vi "Main_Basic.vi"() -> ()   [LabVIEW 2021]
doc: "This template is for the Queued Message Handler design pattern.\n\nThe Event Handling Loop generates messages based on user interface actions.\n\nThe Message Handling Loop processes messages generated by the Event Handling Loop, or by other messages. The messages are string values, so new messages can be added easily to the Message Cases case structure in the Message Handling Loop. Each message cluster can also provide an optional value for Message Data, which is a variant that can be converted to whatever message-specific data is required."
uses:
  Controls/Status Lights.ctl
  Controls/UI Data.ctl
  Controls/Timer Actions.ctl
  support/Message Queue/Enqueue Message (Single).vi
  <vilib>/Utility/error.llb/Error Cluster From Error Code.vi
  <vilib>/ErrorRing/Error Ring.xnode
  support/Message Queue/Message Queue.lvlib
  support/User Event - Stop/User Event - Stop.lvlib
panel:
  out "Sampling Active":bool=TRUE
  out "Pressure":dbl(knob) scale=0.0..10.0
  out "Pressure (Bar)":dbl
  out "Sampling State":string
  in  "Start Pressure Logging":bool
  out "Speed Indicator":dbl
  in  "Release Brake":bool
  in  "Retract":bool
  out "Status":T1
  in  "Speed (v)":dbl(knob) scale=0.0..5.0
  out "Status Message":string
  in  "Extend":bool
  in  "Apply Brake":bool
  in  "Exit":bool
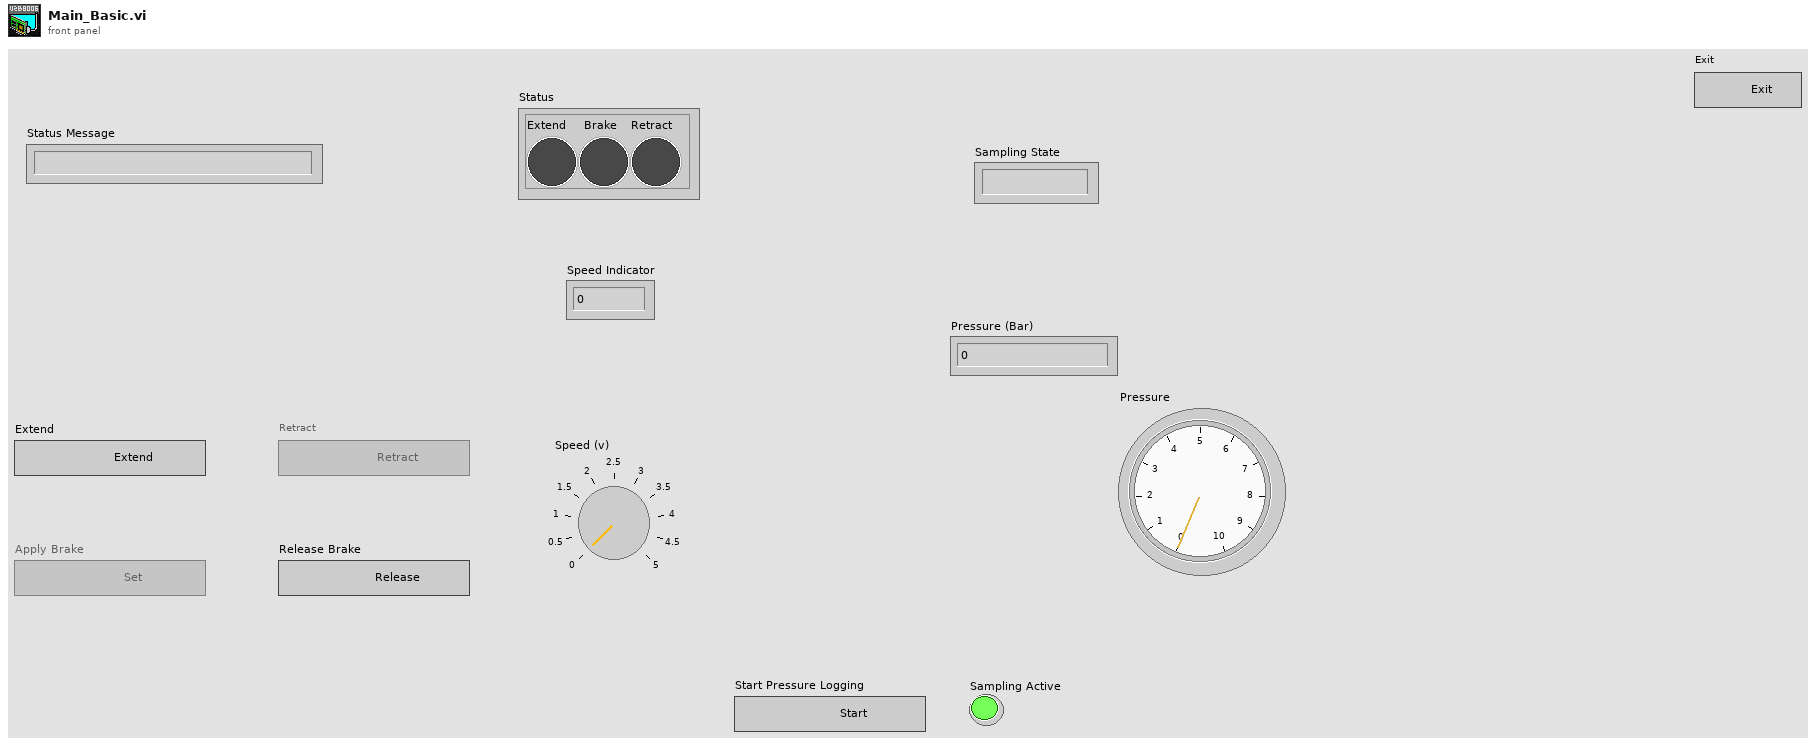
[diagram p1: front panel]
types:
  T1 = typedef "Status Lights.ctl" = cluster{"Extend":bool, "Brake":bool, "Retract":bool}
  T2 = typedef "UI Data.ctl" = cluster{"Sampling State":string, "Status Message":string, "Speed":dbl, "Pressure":dbl, "Apply Brake Ref":refnum<vi>, "Release Brake Ref":refnum<vi>, "Extend Ref":refnum<vi>, "Retract Ref":refnum<vi>, "Pressure Ref":refnum<vi>, "Data Display Ref":refnum<vi>, "Exit Button Ref":refnum<vi>, "Status":T1}
  T3 = typedef "Message Queue.lvlib/All Message Queues.ctl" = cluster{"UI":refnum<queue>}
  T4 = typedef "DAQ Refnums.ctl" = cluster{"Direction Ref":refnum<k21>, "Brake Ref":refnum<k21>, "Speed Ref":refnum<k21>, "Pressure Ref":refnum<k21>}
  T5 = typedef "Timer Actions.ctl" = enum16{"Start Timer", "Restart Timer", "Check Timer", "Pause Timer", "Reset Timer", "Exit Timer"}
  T6 = enum8{"Enabled", "Disabled", "Disabled and Grayed Out"}
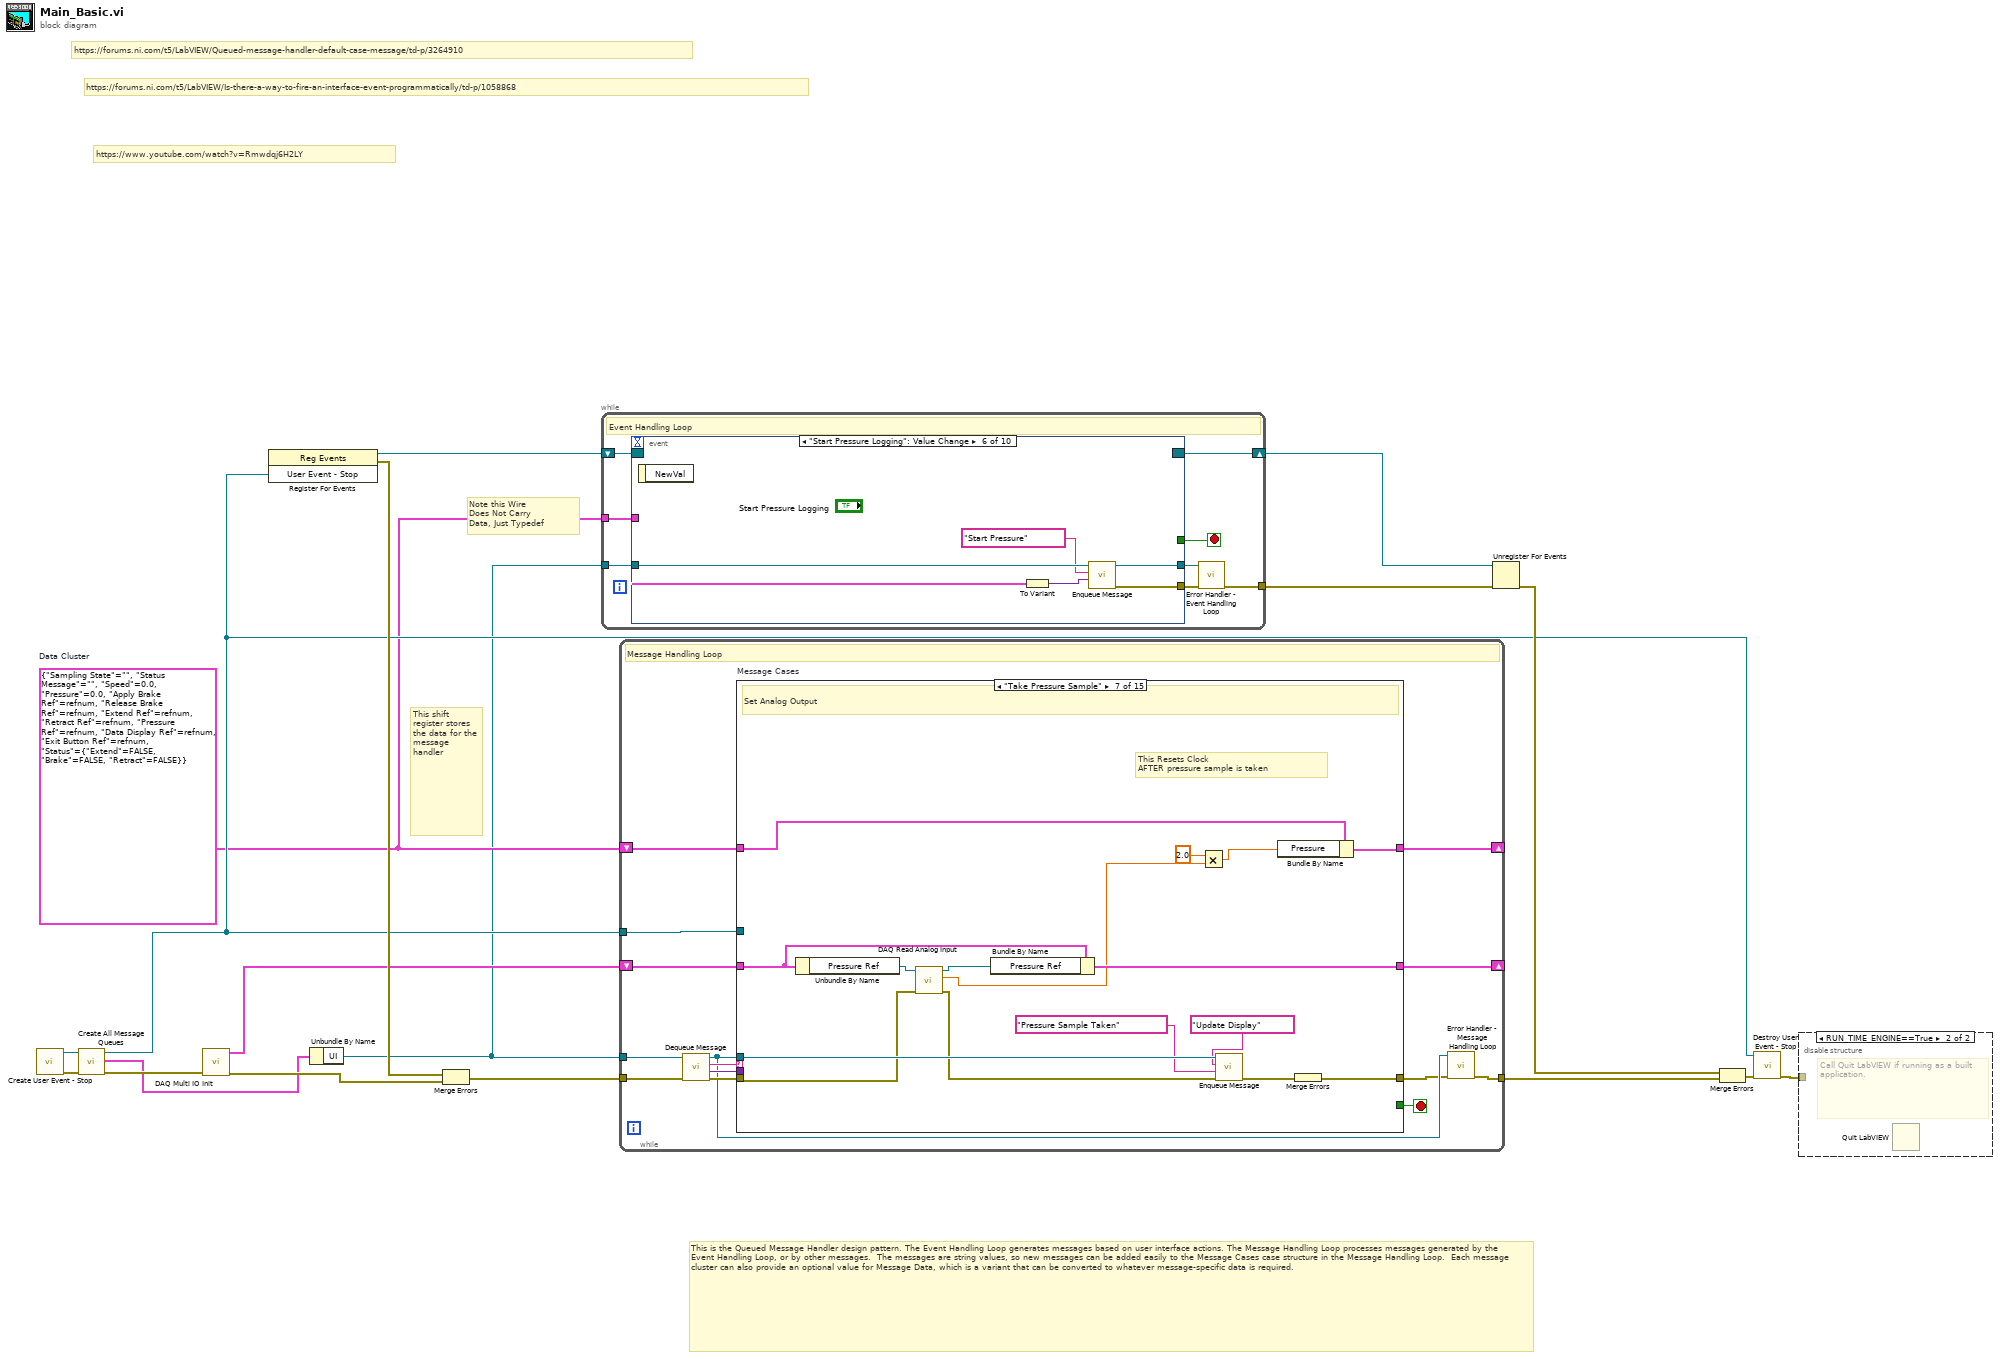
[diagram p0: block diagram]
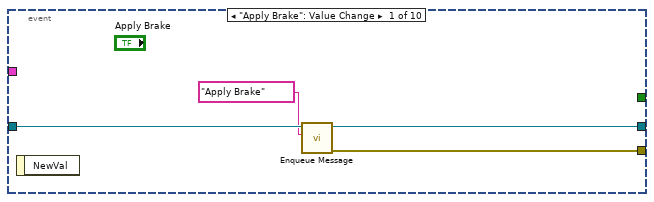
[diagram p3: hidden frame]
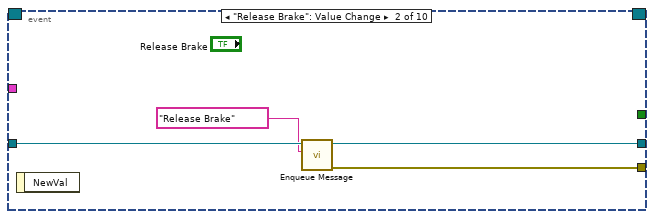
[diagram p4: hidden frame]
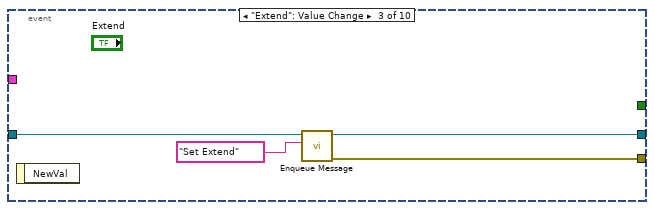
[diagram p5: hidden frame]
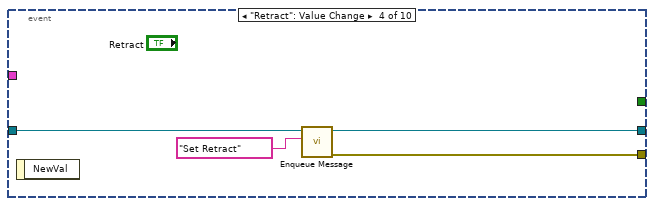
[diagram p6: hidden frame]
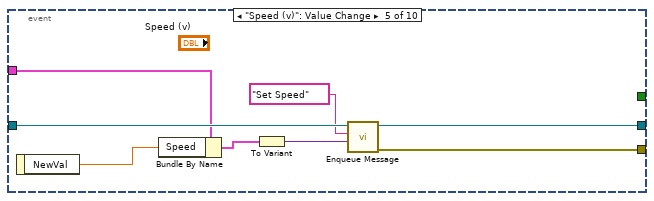
[diagram p7: hidden frame]
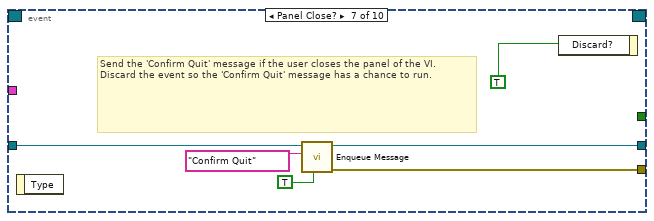
[diagram p8: hidden frame]
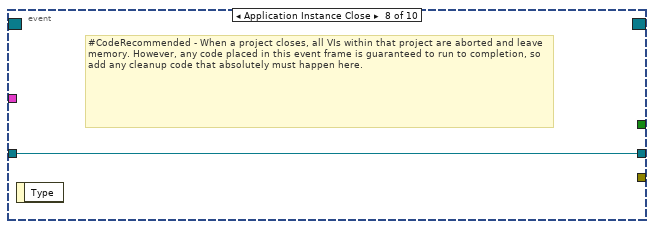
[diagram p9: hidden frame]
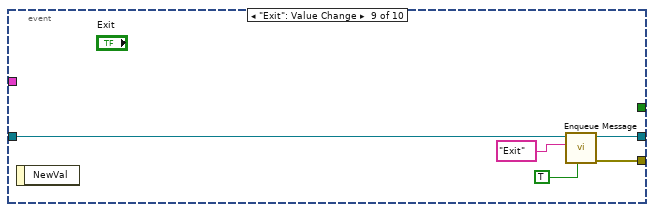
[diagram p10: hidden frame]
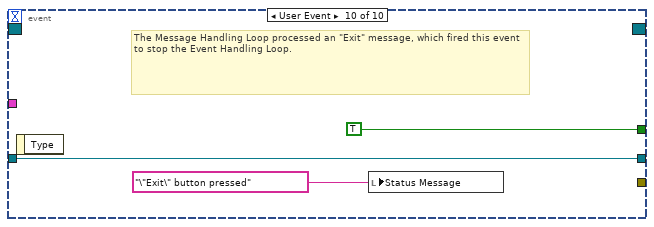
[diagram p11: hidden frame]
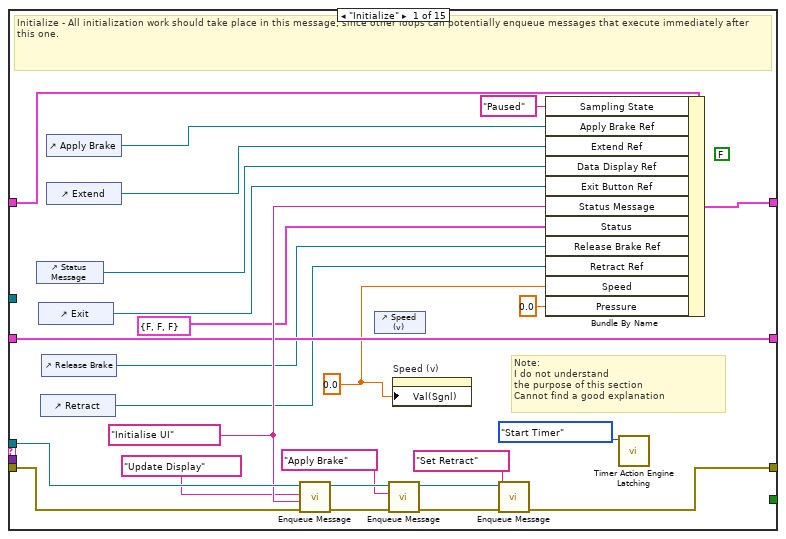
[diagram p12: hidden frame]
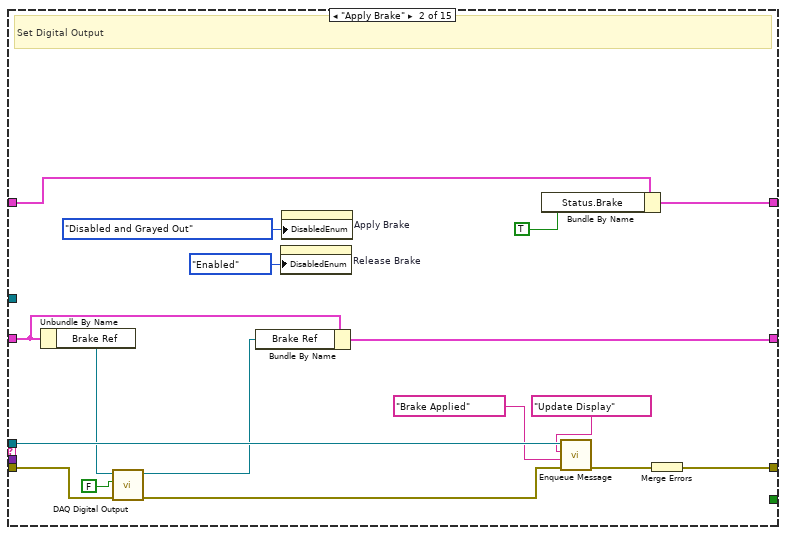
[diagram p13: hidden frame]
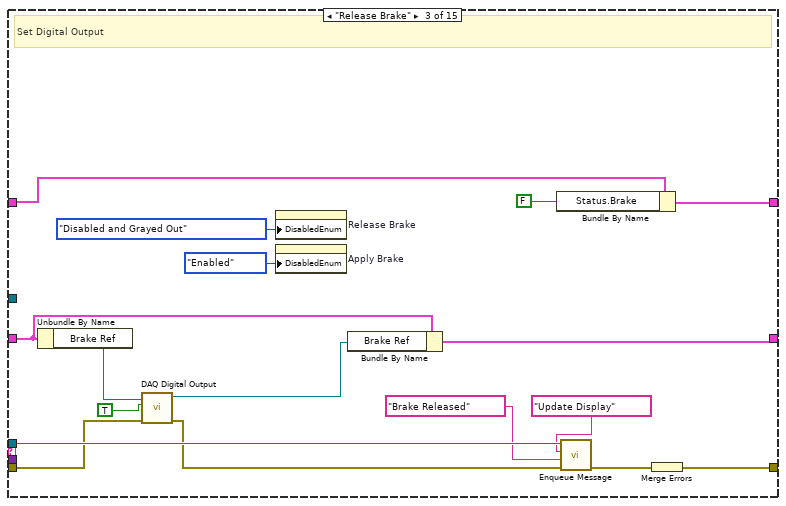
[diagram p14: hidden frame]
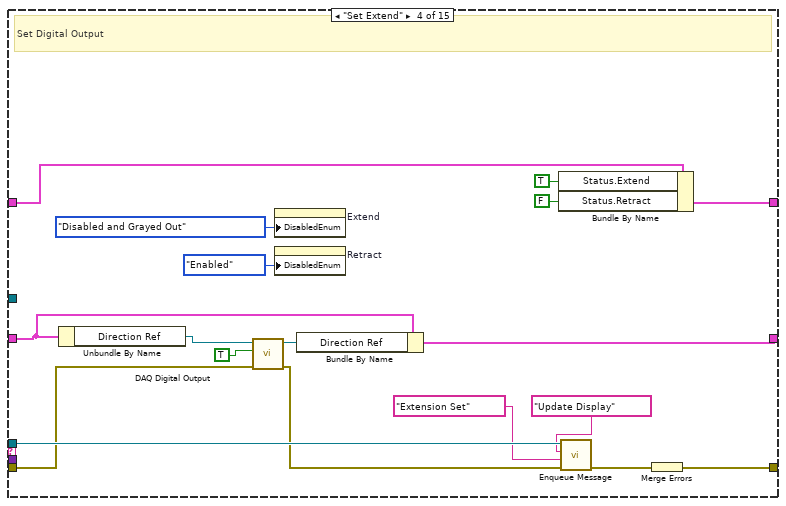
[diagram p15: hidden frame]
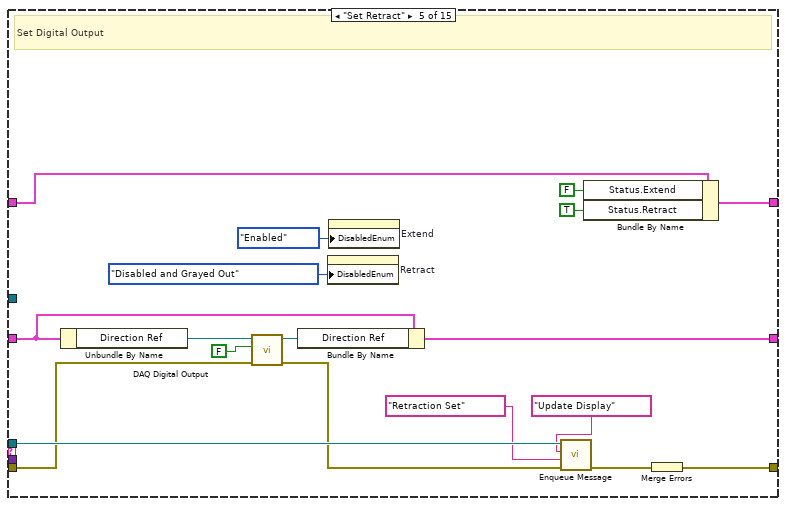
[diagram p16: hidden frame]
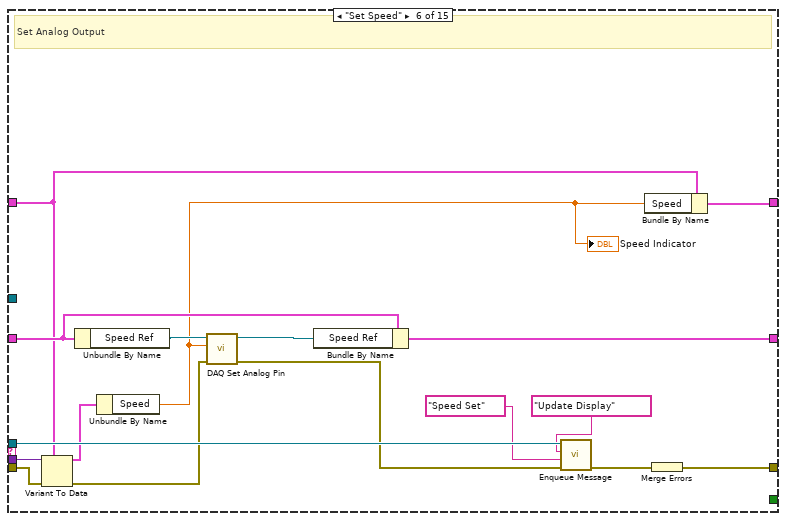
[diagram p17: hidden frame]
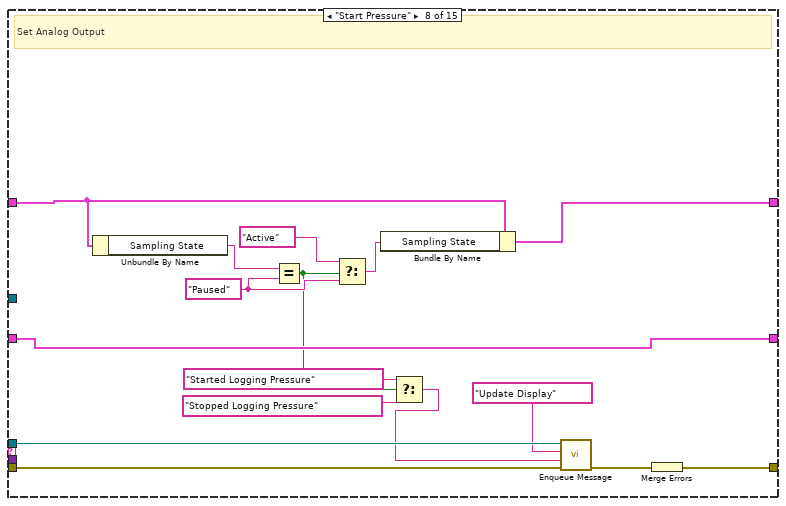
[diagram p18: hidden frame]
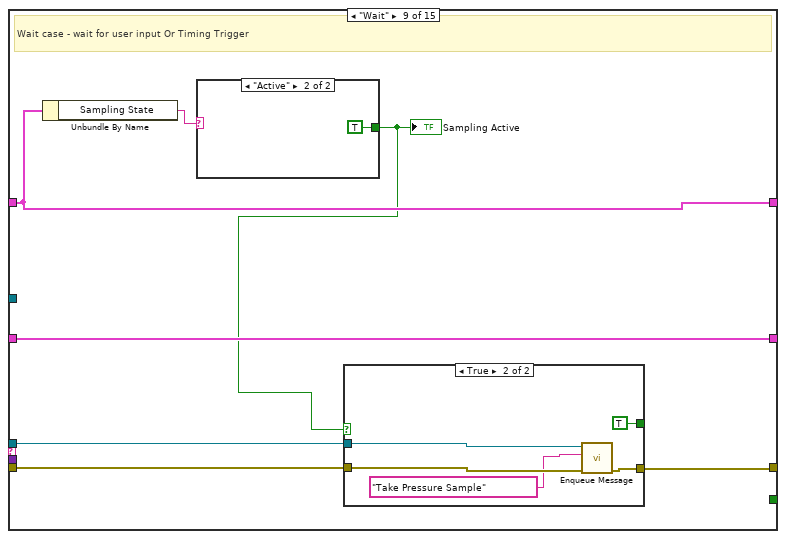
[diagram p19: hidden frame]
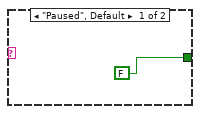
[diagram p20: hidden frame]
diagram:
  w2 = T2 {"Sampling State"="", "Status Message"="", "Speed"=0.0, "Pressure"=0.0, "Apply Brake Ref"=refnum, "Release Brake Ref"=refnum, "Extend Ref"=refnum, "Retract Ref"=refnum, "Pressure Ref"=refnum, "Data Display Ref"=refnum, "Exit Button Ref"=refnum, "Status"={"Extend"=FALSE, "Brake"=FALSE, "Retract"=FALSE}}  # Data Cluster
  # "Note this Wire\nDoes Not Carry\nData, Just Typedef"
  # "https://www.youtube.com/watch?v=Rmwdqj6H2LY"
  # "https://forums.ni.com/t5/LabVIEW/Is-there-a-way-to-fire-an-interface-event-programmatically/td-p/1058868"
  # "https://forums.ni.com/t5/LabVIEW/Queued-message-handler-default-case-message/td-p/3264910"
  # "This is the Queued Message Handler design pattern. The Event Handling Loop generates messages based on user interface actions. The Message Handling Loop processes messages generated by the Event Handling Loop, or by other messages.  The messages are string values, so new messages can be added easily to the Message Cases case structure in the Message Handling Loop.  Each message cluster can also provide an optional value for Message Data, which is a variant that can be converted to whatever message-specific data is required."
  # "This shift register stores the data for the message handler"
  n1 = call "Create User Event - Stop.vi"() -> ("error out"=w17:errorcluster, "User Event - Stop"=w6:refnum<user-event>)  [unwired: 10 in]
  n2 = call "Create All Message Queues.vi"("error in (no error)"=w17) -> ("error out"=w5:errorcluster, "Message Queues out"=w3:T3)  [unwired: 9 in]
  n3 = call "DAQ Multi IO Init.vi"("error in"=w5) -> ("error out"=w4:errorcluster, "DAQ Ref Cluster"=w7:T4)  [unwired: 9 in]
  n4 = register-events(w6) -> (reference out=w11:refnum<event-registration>, error out=w10:errorcluster)  [unwired: 2 in]
  n5 = Unbundle By Name(w3) -> ("UI"=w1:refnum<queue>)
  n6 = Merge Errors(w10, w4) -> (w8:errorcluster)
  n7 = while {
    tunnel: w1 -> [w25]
    shift-right: [w23] -> w14
    shift-left: w11 -> [w24]
    tunnel: [w19] -> w12
    tunnel: w2 -> [w18]
    stop <- w21 stop-if-true
    # "Event Handling Loop"
    n8 = event shown="[5] \"Start Pressure Logging\": Value Change" {
      selector: w24 -> [_ _ _ _ _ _ _ _ _ _]
      dyn-events: [_ _ _ _ _ _ _ _ _ _] -> w23
      timeout: _ -> [_ _ _ _ _ _ _ _ _ _]
      tunnel: [_ _ _ _ _ _ _ _ _ TRUE ("Discard?")] -> w21
      tunnel: w25 -> [w29 w33 w37 w41 w49 w53 w60 w62 w67 w70]
      tunnel: [w26 w30 w34 w38 w46 w54 w59 _ w66 _] -> w22
      tunnel: [w28 w32 w36 w40 w48 w55 w58 w62 w65 w70] -> w20
      tunnel: w18 -> [_ _ _ _ w42 w50 _ _ _ _]
      event "Apply Brake": Value Change {
        n9 = event-data() -> ()  [unwired: 1 in, 1 out]
        n10 = call-poly "Enqueue Message.vi"("Message"="Apply Brake", "Message Queue"=w29) -> ("error out"=w26:errorcluster, "dup Message Queue"=w28:refnum<queue>)  [unwired: 8 in]
      }
      event "Release Brake": Value Change {
        n11 = event-data() -> ()  [unwired: 1 in, 1 out]
        n12 = call-poly "Enqueue Message.vi"("Message"="Release Brake", "Message Queue"=w33) -> ("error out"=w30:errorcluster, "dup Message Queue"=w32:refnum<queue>)  [unwired: 8 in]
      }
      event "Extend": Value Change {
        n13 = event-data() -> ()  [unwired: 1 in, 1 out]
        n14 = call-poly "Enqueue Message.vi"("Message"="Set Extend", "Message Queue"=w37) -> ("error out"=w34:errorcluster, "dup Message Queue"=w36:refnum<queue>)  [unwired: 8 in]
      }
      event "Retract": Value Change {
        n15 = event-data() -> ()  [unwired: 1 in, 1 out]
        n16 = call-poly "Enqueue Message.vi"("Message"="Set Retract", "Message Queue"=w41) -> ("error out"=w38:errorcluster, "dup Message Queue"=w40:refnum<queue>)  [unwired: 8 in]
      }
      event "Speed (v)": Value Change {
        n17 = event-data() -> ("NewVal"=w44:dbl)  [unwired: 1 in]
        n18 = Bundle By Name(cluster=w42, "Speed"=w44) -> (w43:T2)
        n19 = To Variant(anything=w43) -> (Variant=w45:variant)
        n20 = call-poly "Enqueue Message.vi"("Message Data"=w45, "Message"="Set Speed", "Message Queue"=w49) -> ("error out"=w46:errorcluster, "dup Message Queue"=w48:refnum<queue>)  [unwired: 7 in]
      }
      event "Start Pressure Logging": Value Change {
        n21 = event-data() -> ()  [unwired: 1 in, 1 out]
        n22 = To Variant(anything=w50) -> (Variant=w51:variant)
        n23 = call-poly "Enqueue Message.vi"("Message Data"=w51, "Message"="Start Pressure", "Message Queue"=w53) -> ("error out"=w54:errorcluster, "dup Message Queue"=w55:refnum<queue>)  [unwired: 7 in]
      }
      event Panel Close? {
        # "Send the 'Confirm Quit' message if the user closes the panel of the VI. Discard the event so the 'Confirm Quit' message has a chance to run."
        n24 = event-data() -> ()  [unwired: 1 in, 1 out]
        n25 = call-poly "Enqueue Message.vi"("Priority Message? (F)"=TRUE, "Message"="Confirm Quit", "Message Queue"=w60) -> ("error out"=w59:errorcluster, "dup Message Queue"=w58:refnum<queue>)  [unwired: 7 in]
        n26 = event-data("Discard?"=TRUE) -> ()  [unwired: 1 in, 1 out]
      }
      event Application Instance Close {
        # "#CodeRecommended - When a project closes, all VIs within that project are aborted and leave memory. However, any code placed in this event frame is guaranteed to run to completion, so add any cleanup code that absolutely must happen here."
        n27 = event-data() -> ()  [unwired: 1 in, 1 out]
      }
      event "Exit": Value Change {
        n28 = event-data() -> ()  [unwired: 1 in, 1 out]
        n29 = call-poly "Enqueue Message.vi"("Priority Message? (F)"=TRUE, "Message"="Exit", "Message Queue"=w67) -> ("error out"=w66:errorcluster, "dup Message Queue"=w65:refnum<queue>)  [unwired: 7 in]
      }
      event User Event {
        # "The Message Handling Loop processed an \"Exit\" message, which fired this event to stop the Event Handling Loop."
        n30 = event-data() -> ()  [unwired: 1 in, 1 out]
        n31 = local write "Status Message"("\"Exit\" button pressed" ("VI Stopped")) -> ()
      }
    }
    n32 = call "Error Handler - Event Handling Loop.vi"("error in (no error)"=w22, "Message Queue"=w20) -> ("dup error in"=w19:errorcluster)  [unwired: 8 in, 1 out]
  }
  n33 = while {
    tunnel: w1 -> [w78]
    shift-right: [w73] -> _
    shift-left: w2 -> [w84]
    tunnel: w6 -> [w82]
    tunnel: [w76] -> w9
    tunnel: w8 -> [w74]
    shift-right: [w71] -> _
    shift-left: w7 -> [w72]
    stop <- w83 stop-if-true
    # "Message Handling Loop"
    n34 = call "Dequeue Message.vi"("error in (no error)"=w74, "Message Queue"=w78) -> ("error out"=w81:errorcluster, "Message Data"=w79:variant, "Message"=w80:string, "dup Message Queue"=w77:refnum<queue>)  [unwired: 6 in]
    n35 = case "Message Cases" shown="\"Take Pressure Sample\"" w80 {
      selector: w80 -> [_ _ _ _ _ _ _ _ _ _ _ _ _ _ w302]
      tunnel: w77 -> [w105 w124 w141 w159 w177 w194 w210 w226 w232 w246 _ w270 _ w300 _]
      tunnel: w81 -> [w109 w122 w139 w157 w175 w185 w197 w218 w234 w252 w266 w274 w278 w295 _]
      tunnel: [w90 w126 w143 w161 w179 w196 w212 w228 w233 w258 w260 w272 w276 w297 w303] -> w75
      tunnel: w84 -> [w97 w116 w127 w144 w164 w182 w205 w219 w231 w254 w265 w273 w277 w299 w304]
      tunnel: [w108 w119 w136 w154 w172 w181 w204 w221 w231 w254 w265 w273 w277 w299 w304] -> w73
      tunnel: [_ _ _ _ _ _ _ _ _ _ _ _ _ TRUE _] -> w83
      tunnel: w79 -> [_ _ _ _ _ w186 _ _ _ w253 w264 _ _ w292 _]
      tunnel: w82 -> [_ _ _ _ _ _ _ _ _ _ _ _ _ w296 _]
      tunnel: w72 -> [w101 w114 w131 w150 w168 w191 w207 w222 w235 w256 w259 w267 w275 w284 w301]
      tunnel: [w101 w113 w130 w149 w167 w190 w206 w222 w235 w256 w259 w267 w275 w285 w301] -> w71
      frame "Initialize" {
        (unwired) FALSE ("Clock Output")
        w98 = 0.0 ("Speed")
        w104 = "Initialise UI" ("Initial Message")
        # "Note:\nI do not understand\nthe purpose of this section\nCannot find a good explanation"
        # "Initialize - All initialization work should take place in this message, since other loops can potentially enqueue messages that execute immediately after this one."
        n36 = control-ref of="Status Message"() -> (w107:refnum<vi>)
        n37 = control-ref of="Exit"() -> (w106:refnum<vi>)
        n38 = control-ref of="Retract"() -> (w99:refnum<vi>)
        n39 = control-ref of="Release Brake"() -> (w100:refnum<vi>)
        n40 = control-ref of="Apply Brake"() -> (w103:refnum<vi>)
        n41 = control-ref of="Extend"() -> (w96:refnum<vi>)
        n42 = call-poly "Enqueue Message.vi"("error in (no error)"=w109, "Message Data"=w104, "Message"="Update Display", "Message Queue"=w105) -> ("error out"=w94:errorcluster, "dup Message Queue"=w93:refnum<queue>)  [unwired: 6 in]
        n43 = control-ref of="Speed (v)"() -> ()  [unwired: 1 out]
        n44 = call-poly "Enqueue Message.vi"("error in (no error)"=w94, "Message"="Apply Brake", "Message Queue"=w93) -> ("error out"=w91:errorcluster, "dup Message Queue"=w89:refnum<queue>)  [unwired: 7 in]
        n45 = property on="Speed (v)" class="Knob (strict)"("Val(Sgnl)"=w98) -> ()  [unwired: 2 in, 2 out]
        n46 = call-poly "Enqueue Message.vi"("error in (no error)"=w91, "Message"="Set Retract", "Message Queue"=w89) -> ("error out"=w90:errorcluster)  [unwired: 7 in, 1 out]
        n47 = Bundle By Name(cluster=w97, "Sampling State"="Paused", "Apply Brake Ref"=w103, "Extend Ref"=w96, "Data Display Ref"=w107, "Exit Button Ref"=w106, "Status Message"=w104, "Status"=T1 {"Extend"=FALSE, "Brake"=FALSE, "Retract"=FALSE}, "Release Brake Ref"=w100, "Retract Ref"=w99, "Speed"=w98, "Pressure"=0.0) -> (w108:T2)
        n48 = call "Timer Action Engine Latching.vi"("Action"=Timer_Actions."Start Timer") -> ()  [unwired: 7 in, 4 out]
      }
      frame "Apply Brake" {
        # "Set Digital Output"
        n49 = Unbundle By Name(w114) -> ("Brake Ref"=w115:refnum<k21>)
        n50 = call "DAQ Digital Output.vi"("error in"=w122, "data"=FALSE, "task/channels in"=w115) -> ("error out"=w121:errorcluster, "task out"=w112:refnum<k21>)  [unwired: 6 in, 1 out]
        n51 = Bundle By Name(cluster=w114, "Brake Ref"=w112) -> (w113:T4)
        n52 = property on="Release Brake" class="Bool"("DisabledEnum"=T6."Enabled" ("Disabled")) -> ()  [unwired: 2 in, 2 out]
        n53 = property on="Apply Brake" class="Bool"("DisabledEnum"=T6."Disabled and Grayed Out" ("Disabled")) -> ()  [unwired: 2 in, 2 out]
        n54 = Bundle By Name(cluster=w116, "Status.Brake"=TRUE) -> (w119:T2)
        n55 = call-poly "Enqueue Message.vi"("error in (no error)"=w121, "Message Data"="Brake Applied" ("\"Do Something\" button pressed"), "Message"="Update Display", "Message Queue"=w124) -> ("error out"=w125:errorcluster)  [unwired: 6 in, 1 out]
        n56 = Merge Errors(w125) -> (w126:errorcluster)
      }
      frame "Release Brake" {
        # "Set Digital Output"
        n57 = Unbundle By Name(w131) -> ("Brake Ref"=w133:refnum<k21>)
        n58 = call "DAQ Digital Output.vi"("error in"=w139, "data"=TRUE, "task/channels in"=w133) -> ("error out"=w138:errorcluster, "task out"=w132:refnum<k21>)  [unwired: 6 in, 1 out]
        n59 = property on="Release Brake" class="Bool"("DisabledEnum"=T6."Disabled and Grayed Out" ("Disabled")) -> ()  [unwired: 2 in, 2 out]
        n60 = property on="Apply Brake" class="Bool"("DisabledEnum"=T6."Enabled" ("Disabled")) -> ()  [unwired: 2 in, 2 out]
        n61 = Bundle By Name(cluster=w131, "Brake Ref"=w132) -> (w130:T4)
        n62 = Bundle By Name(cluster=w127, "Status.Brake"=FALSE ("Boolean")) -> (w136:T2)
        n63 = call-poly "Enqueue Message.vi"("error in (no error)"=w138, "Message Data"="Brake Released" ("\"Do Something\" button pressed"), "Message"="Update Display", "Message Queue"=w141) -> ("error out"=w142:errorcluster)  [unwired: 6 in, 1 out]
        n64 = Merge Errors(w142) -> (w143:errorcluster)
      }
      frame "Set Extend" {
        # "Set Digital Output"
        n65 = Unbundle By Name(w150) -> ("Direction Ref"=w152:refnum<k21>)
        n66 = call "DAQ Digital Output.vi"("error in"=w157, "data"=TRUE, "task/channels in"=w152) -> ("error out"=w156:errorcluster, "task out"=w151:refnum<k21>)  [unwired: 6 in, 1 out]
        n67 = property on="Extend" class="Bool"("DisabledEnum"=T6."Disabled and Grayed Out" ("Disabled")) -> ()  [unwired: 2 in, 2 out]
        n68 = property on="Retract" class="Bool"("DisabledEnum"=T6."Enabled" ("Disabled")) -> ()  [unwired: 2 in, 2 out]
        n69 = Bundle By Name(cluster=w150, "Direction Ref"=w151) -> (w149:T4)
        n70 = Bundle By Name(cluster=w144, "Status.Extend"=TRUE ("Status.Retract"), "Status.Retract"=FALSE ("Status.Extend")) -> (w154:T2)
        n71 = call-poly "Enqueue Message.vi"("error in (no error)"=w156, "Message Data"="Extension Set" ("\"Do Something\" button pressed"), "Message"="Update Display", "Message Queue"=w159) -> ("error out"=w160:errorcluster)  [unwired: 6 in, 1 out]
        n72 = Merge Errors(w160) -> (w161:errorcluster)
      }
      frame "Set Retract" {
        # "Set Digital Output"
        n73 = Unbundle By Name(w168) -> ("Direction Ref"=w170:refnum<k21>)
        n74 = call "DAQ Digital Output.vi"("error in"=w175, "data"=FALSE, "task/channels in"=w170) -> ("error out"=w174:errorcluster, "task out"=w169:refnum<k21>)  [unwired: 6 in, 1 out]
        n75 = Bundle By Name(cluster=w168, "Direction Ref"=w169) -> (w167:T4)
        n76 = property on="Retract" class="Bool"("DisabledEnum"=T6."Disabled and Grayed Out" ("Disabled")) -> ()  [unwired: 2 in, 2 out]
        n77 = property on="Extend" class="Bool"("DisabledEnum"=T6."Enabled" ("Disabled")) -> ()  [unwired: 2 in, 2 out]
        n78 = call-poly "Enqueue Message.vi"("error in (no error)"=w174, "Message Data"="Retraction Set" ("\"Do Something\" button pressed"), "Message"="Update Display", "Message Queue"=w177) -> ("error out"=w178:errorcluster)  [unwired: 6 in, 1 out]
        n79 = Bundle By Name(cluster=w164, "Status.Extend"=FALSE ("Status.Retract"), "Status.Retract"=TRUE ("Status.Extend")) -> (w172:T2)
        n80 = Merge Errors(w178) -> (w179:errorcluster)
      }
      frame "Set Speed" {
        # "Set Analog Output"
        n81 = Variant To Data(error in=w185, type=w182, Variant=w186) -> (data=w183:T2, error out=w184:errorcluster)
        n82 = Unbundle By Name(w191) -> ("Speed Ref"=w189:refnum<k21>)
        n83 = Unbundle By Name(w183) -> ("Speed"=w180:dbl)
        "Speed Indicator" <- w180
        n84 = call "DAQ Set Analog Pin.vi"("error in"=w184, "Voltage"=w180, "task/channels in"=w189) -> ("error out"=w187:errorcluster, "task out"=w188:refnum<k21>)  [unwired: 6 in, 1 out]
        n85 = Bundle By Name(cluster=w191, "Speed Ref"=w188) -> (w190:T4)
        n86 = call-poly "Enqueue Message.vi"("error in (no error)"=w187, "Message Data"="Speed Set" ("\"Do Something\" button pressed"), "Message"="Update Display", "Message Queue"=w194) -> ("error out"=w195:errorcluster)  [unwired: 6 in, 1 out]
        n87 = Bundle By Name(cluster=w182, "Speed"=w180) -> (w181:T2)
        n88 = Merge Errors(w195) -> (w196:errorcluster)
      }
      frame "Take Pressure Sample" {
        # "This Resets Clock\nAFTER pressure sample is taken"
        # "Set Analog Output"
        n89 = Unbundle By Name(w207) -> ("Pressure Ref"=w203:refnum<k21>)
        n90 = call "DAQ Read Analog Input.vi"("error in"=w197, "task/channels in"=w203) -> ("error out"=w202:errorcluster, "Voltage"=w200:dbl, "task out"=w201:refnum<k21>)  [unwired: 7 in]
        n91 = Bundle By Name(cluster=w207, "Pressure Ref"=w201) -> (w206:T4)
        n92 = Multiply(x=2.0, y=w200) -> (x*y=w198:dbl)
        n93 = call-poly "Enqueue Message.vi"("error in (no error)"=w202, "Message Data"="Pressure Sample Taken" ("\"Do Something\" button pressed"), "Message"="Update Display", "Message Queue"=w210) -> ("error out"=w211:errorcluster)  [unwired: 6 in, 1 out]
        n94 = Bundle By Name(cluster=w205, "Pressure"=w198) -> (w204:T2)
        n95 = Merge Errors(w211) -> (w212:errorcluster)
      }
      frame "Start Pressure" {
        w216 = "Paused" ("y")
        # "Set Analog Output"
        n96 = Unbundle By Name(w219) -> ("Sampling State"=w217:string)
        n97 = Equal?(x=w217, y=w216) -> (x = y?=w213:bool)
        n98 = Select(t="Active", s=w213, f=w216) -> (s? t:f=w214:string)
        n99 = Bundle By Name(cluster=w219, "Sampling State"=w214) -> (w221:T2)
        n100 = Select(t="Started Logging Pressure" ("Status Message"), s=w213, f="Stopped Logging Pressure") -> (s? t:f=w220:string)
        n101 = call-poly "Enqueue Message.vi"("error in (no error)"=w218, "Message Data"=w220, "Message"="Update Display", "Message Queue"=w226) -> ("error out"=w227:errorcluster)  [unwired: 6 in, 1 out]
        n102 = Merge Errors(w227) -> (w228:errorcluster)
      }
      frame "Wait" {
        # "Wait case - wait for user input Or Timing Trigger"
        n103 = Unbundle By Name(w231) -> ("Sampling State"=w230:string)
        n104 = case shown="\"Active\"" w230 {
          tunnel: [FALSE ("Sampling Active") TRUE ("Sampling Active")] -> w229
          frame "Paused", Default {
          }
          frame "Active" {
          }
        }
        "Sampling Active" <- w229
        n105 = case shown="True" w229 {
          selector: w229 -> [w238 _]
          tunnel: w234 -> [w239 w244]
          tunnel: [w239 w243] -> w233
          tunnel: w232 -> [_ w242]
          tunnel: [w238 TRUE] -> _
          frame False {
          }
          frame True {
            n106 = call-poly "Enqueue Message.vi"("error in (no error)"=w244, "Message"="Take Pressure Sample", "Message Queue"=w242) -> ("error out"=w243:errorcluster)  [unwired: 7 in, 1 out]
          }
        }
      }
      frame "Update Display" {
        # "Update Display - Convert the message data to a string to display in the Data Display indicator."
        n107 = Variant To Data(error in=w252, type="" ("Status Message"), Variant=w253) -> (data=→"Status Message":string, error out=w248:errorcluster)
        n108 = Unbundle By Name(w254) -> ("Status"=→"Status":T1, "Sampling State"=→"Sampling State":string, "Pressure"=→"Pressure (Bar)" →"Pressure":dbl)
        n109 = call-poly "Enqueue Message.vi"("error in (no error)"=w248, "Message"="Wait", "Message Queue"=w246) -> ("error out"=w247:errorcluster)  [unwired: 7 in, 1 out]
        n110 = Merge Errors(w247) -> (w258:errorcluster)
      }
      frame "Error" {
        # "#CodeRecommended - If you ever change the name of this \"Error\" message, you'll need to update the name in the Check Loop Error.vi as well."
        # "#CodeRecommended - Consider creating a system for logging errors in some way. These errors are for notification purposes only. Handling of specific errors should be performed in the message frames that generated the error."
        # "Error - Display an error dialog. This message is sent by the \"Error Handler\" VIs at the end of other loops in this application."
        n111 = Variant To Data(error in=w266, type=errorcluster {"status"=FALSE, "code"=0, "source"=""} ("error constant"), Variant=w264) -> (data=w262:errorcluster, error out=w261:errorcluster)
        n112 = call <vilib>:"Simple Error Handler.vi"("error in (no error)"=w262) -> ()  [unwired: 4 in, 5 out]
        n113 = Merge Errors(w261) -> (w260:errorcluster)
      }
      frame "Confirm Quit" {
        # "#CodeNeeded - If you want to provide an \"Are you sure\" dialog (or some other notification) before the application exits, place that code here. This message is typically sent from a Panel Close? event."
        # "Confirm Quit - Message that can confirm whether or not the user wants to exit the application."
        n114 = call-poly "Enqueue Message.vi"("Priority Message? (F)"=TRUE, "error in (no error)"=w274, "Message"="Exit", "Message Queue"=w270) -> ("error out"=w271:errorcluster)  [unwired: 6 in, 1 out]
        n115 = Merge Errors(w271) -> (w272:errorcluster)
      }
      frame "---Copy This Frame---" {
        # "Duplicate this frame when creating new messages.  Change this comment in the duplicated frame to describe this message."
        n116 = Merge Errors(w278) -> (w276:errorcluster)
      }
      frame "Exit" {
        # "Stop the VI"
        # "Release the message queue reference"
        # "Exit - Exit the application."
        n117 = Release Queue(queue=w300, error in (no error)=w295) -> (error out=w291:errorcluster)  [unwired: 1 in, 2 out]
        n118 = call "Fire User Event - Stop.vi"("User Event - Stop"=w296) -> ("error out"=w280:errorcluster)  [unwired: 10 in]
        n119 = Variant To Data(type=errorcluster {"status"=FALSE, "code"=0, "source"=""} ("error constant"), Variant=w292) -> (data=w293:errorcluster)  [unwired: 1 in, 1 out]
        n120 = Unbundle By Name(w284) -> ("Direction Ref"=w288:refnum<k21>, "Brake Ref"=w287:refnum<k21>, "Speed Ref"=w286:refnum<k21>)
        n121 = call <vilib>:"Simple Error Handler.vi"("error in (no error)"=w293) -> ()  [unwired: 4 in, 5 out]
        n122 = call <vilib>:"DAQmx Clear Task.vi"("task in"=w286, "error in"=w291) -> ("error out"=w290:errorcluster)  [unwired: 13 in]
        n123 = call <vilib>:"DAQmx Clear Task.vi"("task in"=w287, "error in"=w290) -> ("error out"=w289:errorcluster)  [unwired: 13 in]
        n124 = call <vilib>:"DAQmx Clear Task.vi"("task in"=w288, "error in"=w289) -> ("error out"=w279:errorcluster)  [unwired: 13 in]
        n125 = Bundle By Name(cluster=w284, "Direction Ref"=refnum<k21> refnum, "Brake Ref"=refnum<k21> refnum, "Speed Ref"=refnum<k21> refnum) -> (w285:T4)
        n126 = Merge Errors(w280, w279) -> (w297:errorcluster)
      }
      frame Default {
        # "'Default' case only runs if there is a message that isn't defined in any of the other cases.  Output a programming error."
        n127 = xnode "Error Ring"("parameter 0"=w302) -> ("error out"=w303:errorcluster)
      }
    }
    n128 = call "Error Handler - Message Handling Loop.vi"("error in (no error)"=w75, "Message Queue"=w77) -> ("dup error in"=w76:errorcluster)  [unwired: 8 in, 1 out]
  }
  n129 = Unregister For Events(event registration refnum=w14, error in=w12) -> (error out=w15:errorcluster)
  n130 = Merge Errors(w15, w9) -> (w16:errorcluster)
  n131 = call "Destroy User Event - Stop.vi"("error in (no error)"=w16, "User Event - Stop"=w6) -> ("error out"=w13:errorcluster)  [unwired: 9 in]
  n132 = disable-structure shown="RUN_TIME_ENGINE==True" {
    disable-tunnel: w13 -> [_ _]
    frame condition #0 (active) {
    }
    frame condition #1 {
      # "Call Quit LabVIEW if running as a built application."
      n133 = Quit LabVIEW() -> ()  [unwired: 1 in]
    }
  }
